vi "test.vi"() -> ()   [LabVIEW 2021]
panel:
  in  "Boolean":bool
  out "Meter":dbl(knob) scale=0.0..10.0
  out "x+y":dbl
  in  "number 2":dbl
  in  "number 1":dbl
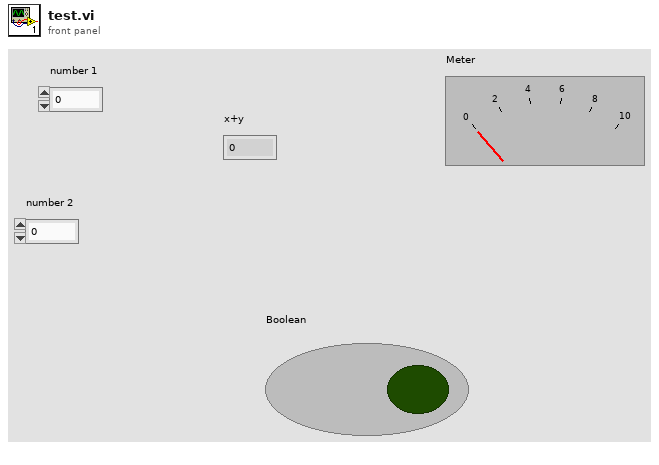
[diagram p1: front panel]
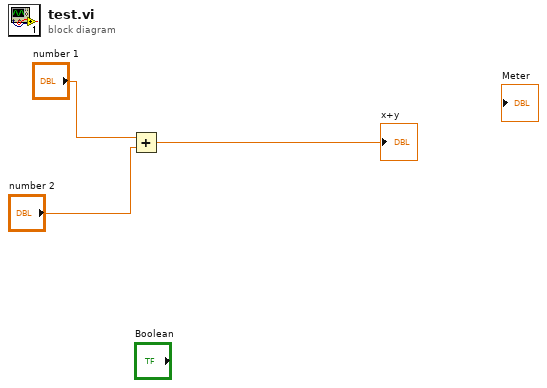
[diagram p0: block diagram]
diagram:
  n1 = Add(x="number 1", y="number 2") -> (x+y=→"x+y":dbl)
